vi "Write outputs.vi"(8 "error in (no error)":errorcluster, 10 "outputs":bool[](array[boolean]), 11 "Power Supply Instrument in":refnum<class "Power Supply Instrument.lvclass">) -> (0 "error out":errorcluster, 3 "Power Supply Instrument out":refnum<class "Power Supply Instrument.lvclass">)   [LabVIEW 2025, in "Power Supply.lvlib" / "Power Supply Instrument.lvclass"]
uses:
  Power Supply Instrument.lvclass
  Power Supply Instrument.lvclass/Power Supply Instrument.ctl
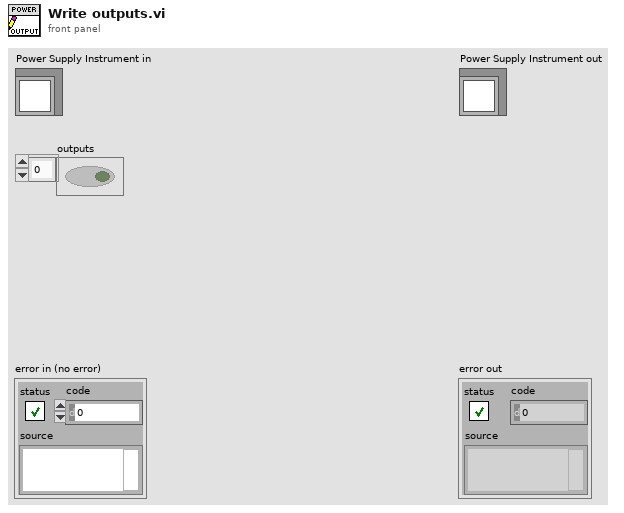
[diagram p1: front panel]
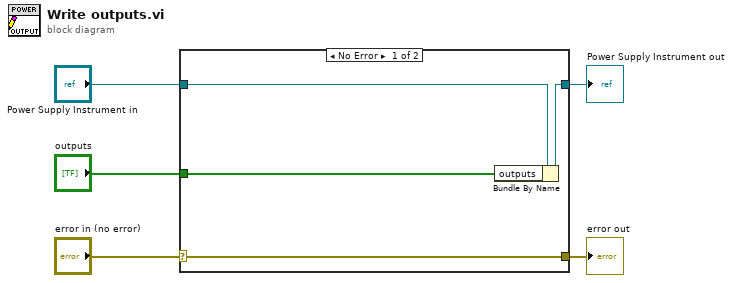
[diagram p0: block diagram]
diagram:
  n1 = case shown="No Error" "error in (no error)" {
    selector: "error in (no error)" -> [w9 w10]
    tunnel: [w9 w10] -> w4
    tunnel: [w7 w11] -> w2
    tunnel: "Power Supply Instrument in" -> [w8 w11]
    tunnel: "outputs" -> [w6 _]
    frame No Error {
      n2 = Bundle By Name(cluster=w8, "outputs"=w6) -> (w7:refnum<class "Power Supply Instrument.lvclass">)
    }
    frame Error {
    }
  }
  "error out" <- w4
  "Power Supply Instrument out" <- w2
